vi "MainPanel.vi"() -> ()   [LabVIEW 2017]
uses:
  <vilib>/Native 3D Graph/xcontrol/3DPC_SurfacePlot.xctl
  <vilib>/Simulation/Scripting/Companion Diagram/SimConfigNode/SimParams.ctl
  <vilib>/Simulation/Scripting/Companion Diagram/SimConfigNode/_simSolvers.ctl
  <vilib>/Simulation/Implementation/Shared/SIMSCR Execution Mode.ctl
  <vilib>/Simulation/Param Hierarchy/Typedefs/SIMPH Param Control Actions.ctl
  <vilib>/addons/Control Design/_Model Construction/Model Typedefs.llb/CD Transfer Function Model (MIMO).ctl
  <vilib>/addons/Control Design/_Model Construction/Model Typedefs.llb/CD General Elements.ctl
  <vilib>/addons/Control Design/_Model Construction/Model Typedefs.llb/CD Transfer Function Model (SISO).ctl
  state.ctl
  Mode.ctl
  <vilib>/Simulation/Implementation/Shared/NILVSim_ParamChanged.vi
  <vilib>/Simulation/Implementation/Shared/NILVSIM_BeginStep.vi
  <vilib>/Simulation/Implementation/Shared/NILVSim_Manager.vi
  <vilib>/Utility/error.llb/Clear Errors.vi
  <vilib>/Simulation/Implementation/Shared/NILVSim_FinalizeModel.vi
  <vilib>/Analysis/coordinate.llb/3D Coordinate Conversion (Scalar).vi
  <vilib>/Simulation/Implementation/Shared/SIM Unbundle Sim Info.vi
  <vilib>/Simulation/Implementation/Shared/NILVSim_Initialize.vi
  <vilib>/Simulation/Utility/Implementation/NILVSim Get Time and IsAcceptedStep.vi
  <vilib>/Simulation/Implementation/Shared/SIMSH Read Queue.vi
  <vilib>/Simulation/Implementation/Shared/NILVSim_GetModelError.vi
  <vilib>/Simulation/Implementation/Shared/SIM Bundle Sim Info.vi
  <vilib>/Simulation/Implementation/XNodeFramework/SimXNode/SimX.xnode
  Tension Control.vi
  <vilib>/Simulation/Scripting/Companion Diagram/SimConfigNode/SimDog.xnode
  <vilib>/Analysis/NI_AALPro.lvlib
  <vilib>/Simulation/Implementation/Shared/NI_SIM_Implementation.lvlib
  <vilib>/addons/Control Design/_Model Construction/NI_LinSys_Model Typedefs.lvlib
panel:
  out "Stretch(mm)":dbl(slide) scale=0.0..10.0
  out "Vs":dbl caption="Vs(m/s)" format="%#_4g"
  in  "delay":dbl=100.0 caption="Interval(ms)"
  out "Count":dbl
  out "Rotation":cluster{"Vs":dbl, "Vx":dbl}(graph)
  in  "Forward":bool
  in  "Backward":bool
  in  "Vx":dbl caption="Vx(m/s)" format="%#_5g"
  in  "Deceleration\n  (m/s^-2)":dbl=1.0
  in  "a":dbl=1.0 caption="Acceleration\n (m/s^-2)"
  in  "Range(m)":dbl=5.0 min=0.0
  in  "Layers":dbl format="%#_4g"
  in  "Reverse":bool
  in  "TLimit":dbl=15.0 caption="Max Force(N)" format="%#_4g"
  in  "Tension":bool
  out "Tension\nChart":cluster{"setpoint":dbl, "output y(t)":dbl}(graph)
  in  "F":dbl(slide)=10.0 caption="Set Tension\n (N)" scale=0.0..40.0
  in  "Auto":bool
  in  "Length(m)":dbl=1.5
  in  "Thick":dbl=0.005 caption="Thickness(m)"
  in  "R":dbl(slide)=0.1 caption="Radius(m)" scale=0.0..0.5
  in  "Gap":dbl=0.1 caption="Gap(m)"
  in  "SetSpeed":dbl=100.0 caption="Set Revolution  \n  (RPM)"
  in  "Rapid":bool
  in  "Set X(m)":dbl min=0.0 max=5.0 format="%#_4g"
  in  "Mode":enum32{"Automatic", "Manual"}(radio)
  in  "Home":bool
  in  "Position(m)":dbl(slide) min=0.0 scale=0.0..5.0 scale format="%#_4g"
  out "Trajectory":refnum<class "Base Datatype.lvclass">[](xcontrol)
  in  "Break":bool
  in  "Power":bool
  # "Motion Control Simulation\nBy Xuehui Zhu"
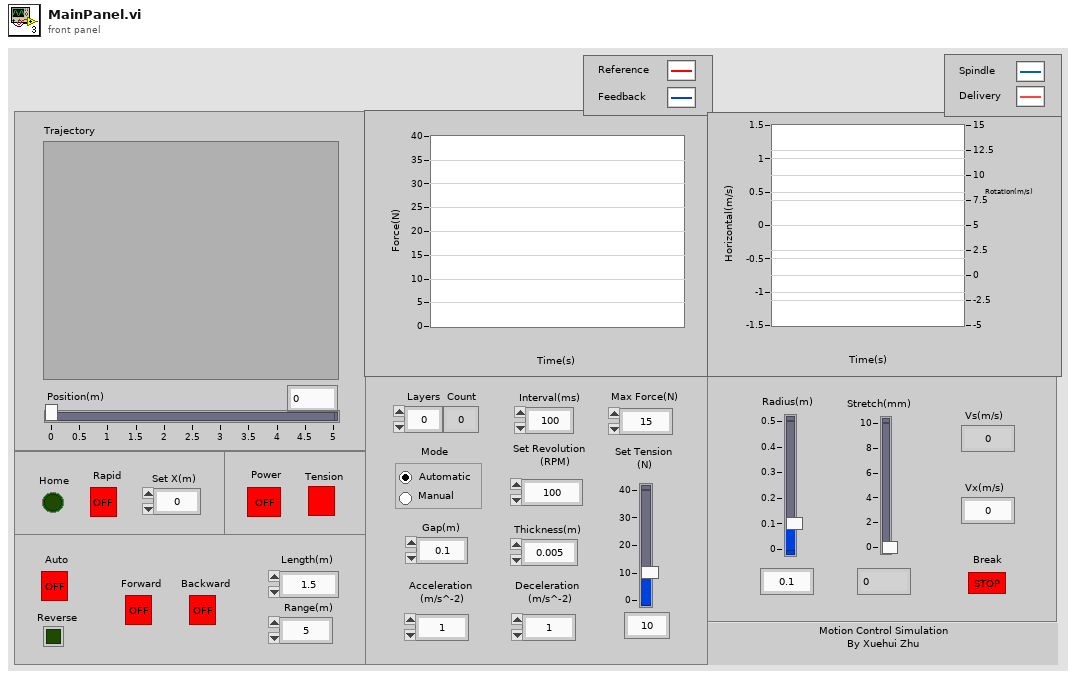
[diagram p1: front panel]
types:
  T1 = enum16{"Simulate to Completion", "Single Time-Step Simulation (Fixed Step Only)"}
  T2 = typedef "SIMSCR Execution Mode.ctl" = enum16{"Simulate to Completion", "Single Time-Step Simulation (Fixed Step Only)"}
  T3 = typedef "SIMPH Param Control Actions.ctl" = enum16{"get params", "set params"}
  T4 = cluster{"proportional gain (Kc)":dbl, "integral time (Ti, min)":dbl, "derivative time (Td, min)":dbl}
  T5 = typedef "NI_LinSys_Model Typedefs.lvlib/CD Transfer Function Model (MIMO).ctl" = cluster{"properties":T6, "transfer function(s)":T7[][]}
  T6 = typedef "NI_LinSys_Model Typedefs.lvlib/CD General Elements.ctl" = cluster{"Model name":string, "Input names":string[], "Output names":string[], "Input Delays":dbl[], "Output Delays":dbl[], "Sampling Time":dbl, "Notes":string}
  T7 = typedef "NI_LinSys_Model Typedefs.lvlib/CD Transfer Function Model (SISO).ctl" = cluster{"Numerator":dbl[], "Denominator":dbl[], "delay":dbl}
  T8 = cluster{"SIMSH Sim Time":dbl, "Gain":cluster{"output":dbl}, "Bundle":cluster{"output cluster":cluster{"setpoint":dbl, "output":dbl}}, "Less?":cluster{"x < y?":bool}, "Transfer Function":cluster{"output y(t)":dbl}, "PID.vi":cluster{"output":dbl}}
  T9 = typedef "SimParams.ctl" = cluster{"Initial Time (s)":dbl, "Final Time (s)":dbl, "Step Size (s)":dbl, "ODE Solver":T10, "Minimum Step Size (s)":dbl, "Maximum Step Size (s)":dbl, "Relative Tolerance":dbl, "Absolute Tolerance":dbl, "Software Timing":bool, "Initial Step Size (s)":dbl, "Automatic Fixed Step Size?":bool, "Automatic Discrete Step Size?":bool, "Discrete Step Size (s)":dbl, "Calculate using Time Step":bool, "Solver Wired?":bool, "Prev.Frm.Expected End":u64, "Prev.Frm.Actual End":u64, "Prev.Frm.Finished Late?":bool, "Prev.Iter.Expected End":u64, "Prev.Iter.Actual End":u64, "Prev.Iter.Finished Late?":bool, "Expected Iteration Start":u64, "Actual Iteration Start":u64, "Expected Frame Start":u64, "Actual Frame Start":u64, "Source Name":string, "Name":string, "Period":i64, "Deadline":i64, "Offset":i64, "Start":i64, "Priority":i32, "Timeout":i32, "Processor":i32, "Mode":enum32{"No Change", "Process missed periods, maintain original phase", "Discard missed periods, maintain original phase", "Process missed periods, ignore original phase", "Discard missed periods, ignore original phase"}, "Wakeup reason":enum32{"Normal", "Aborted", "Asynchronous wakeup", "Timing source error", "Timed loop error", "Timeout"}, "Error":errorcluster, "Source Type":string, "Secondary Source Type":string, "Global End Time":u64, "Global Start Time":u64, "Full Solver Reset":bool, "Execution Mode":T2, "Nan/Inf Check":bool, "Custom Solver Library":string, "Solver Is Variable":bool, "custom solver name":string, "Signal Collection Decimation":u32}
  T10 = typedef "_simSolvers.ctl" = enum16{"Runge-Kutta 1 (Euler)", "Runge-Kutta 2", "Runge-Kutta 3", "Runge-Kutta 4", "Runge-Kutta 23 (variable)", "Runge-Kutta 45 (variable)", "BDF (variable)", "Adams-Moulton (variable)", "Rosenbrock (variable)", "Discrete States Only", "SDIRK 4 (variable)", "Radau 5 (variable)", "Radau 9 (variable)", "Radau 13 (variable)", "Radau [Variable Order] (variable)", "Gear's Method (variable)", "Linearizer", "State Query", "Trim Eval", "Custom Solver"}
  T11 = typedef "state.ctl" = enum16{"Wait", "Forward", "Backward"}
  T12 = typedef "Mode.ctl" = enum32{"Automatic", "Manual"}
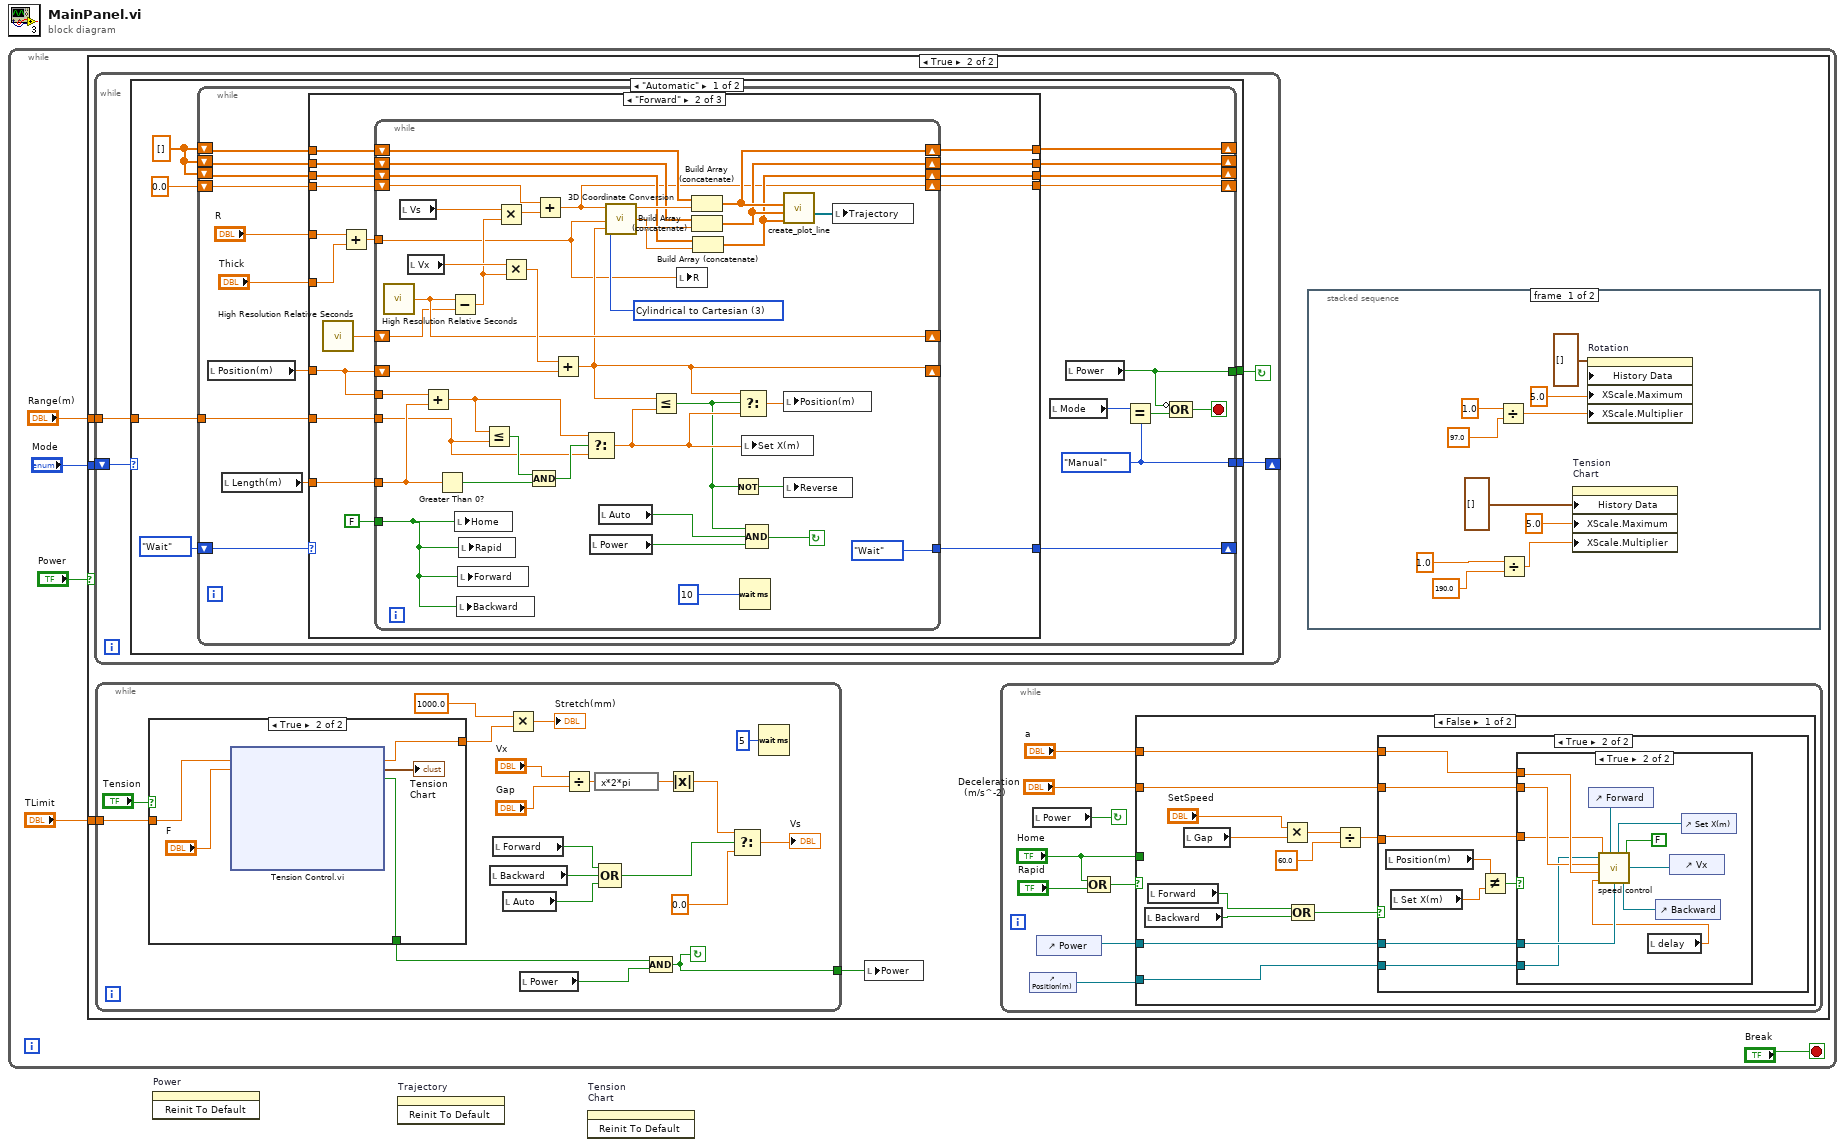
[diagram p0: block diagram]
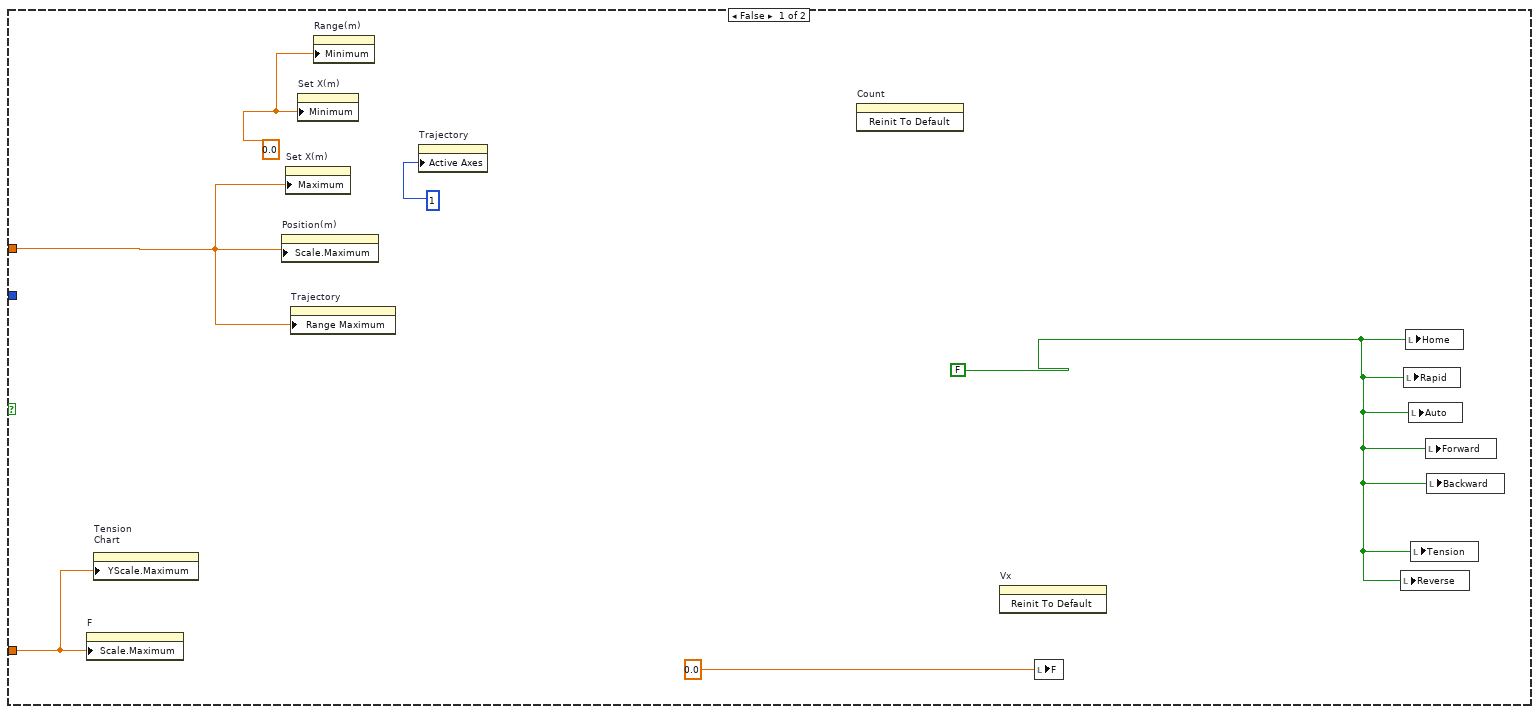
[diagram p2: hidden frame]
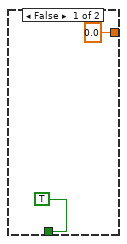
[diagram p3: hidden frame]
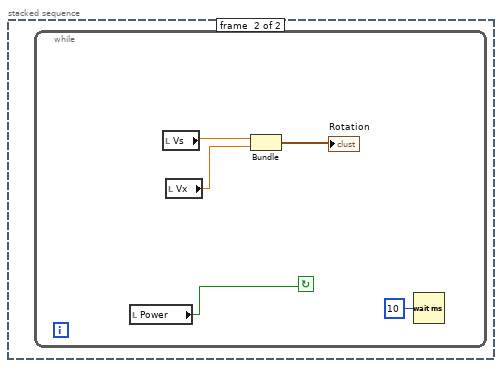
[diagram p4: hidden frame]
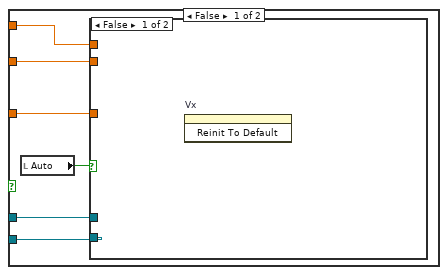
[diagram p5: hidden frame]
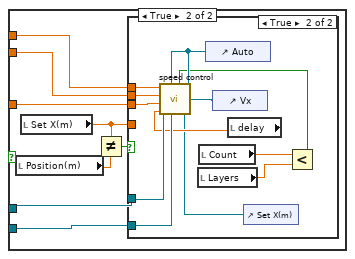
[diagram p6: hidden frame]
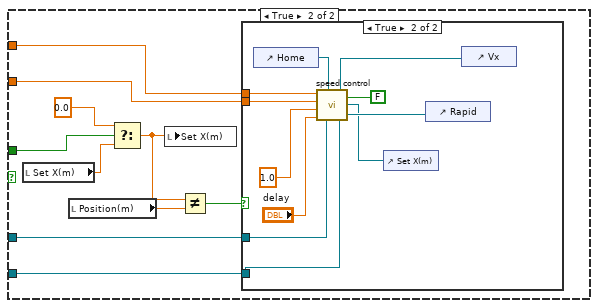
[diagram p9: hidden frame]
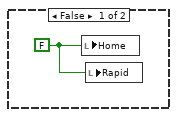
[diagram p10: hidden frame]
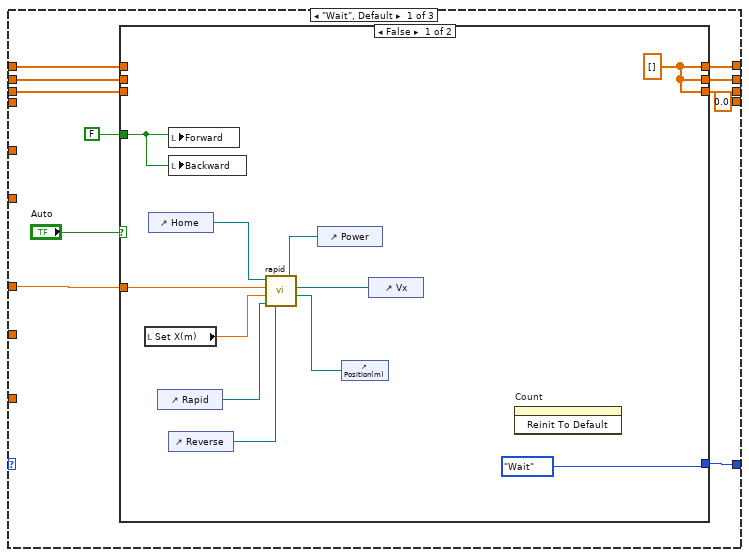
[diagram p11: hidden frame]
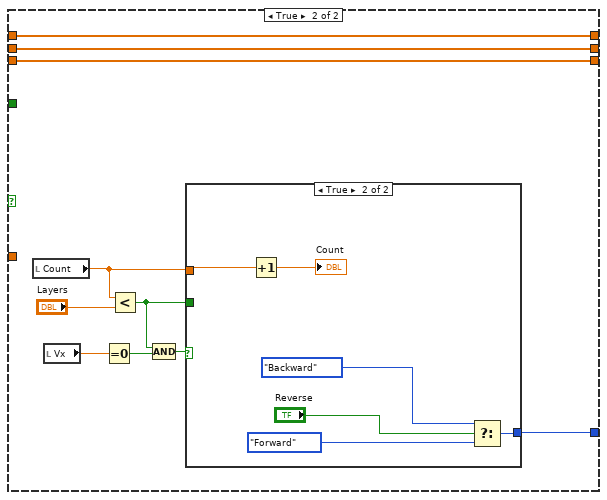
[diagram p12: hidden frame]
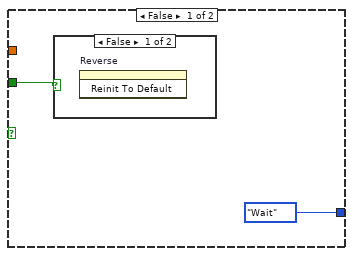
[diagram p13: hidden frame]
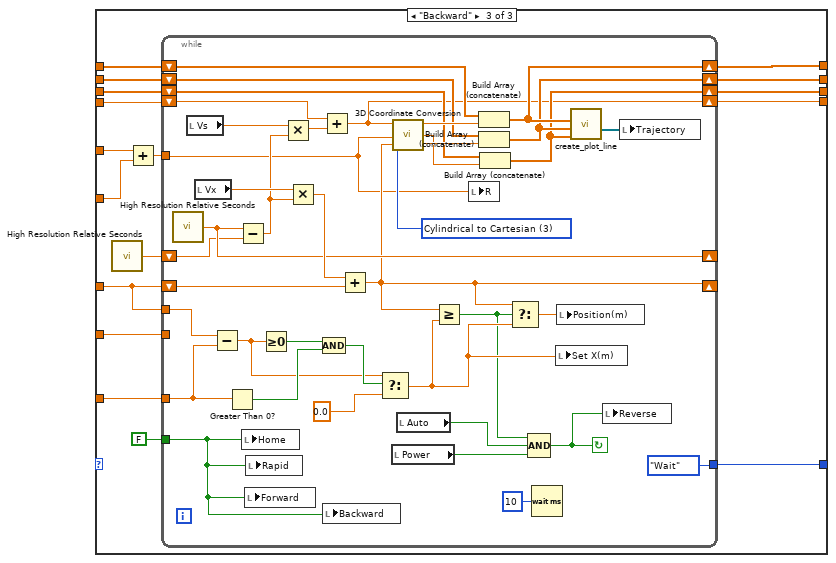
[diagram p15: hidden frame]
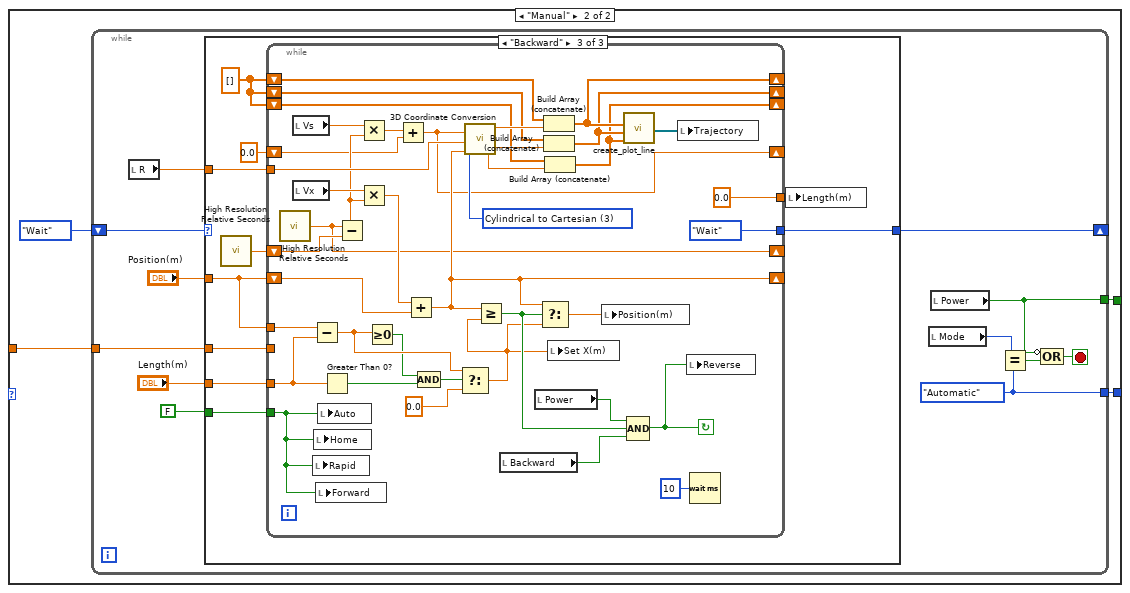
[diagram p16: hidden frame]
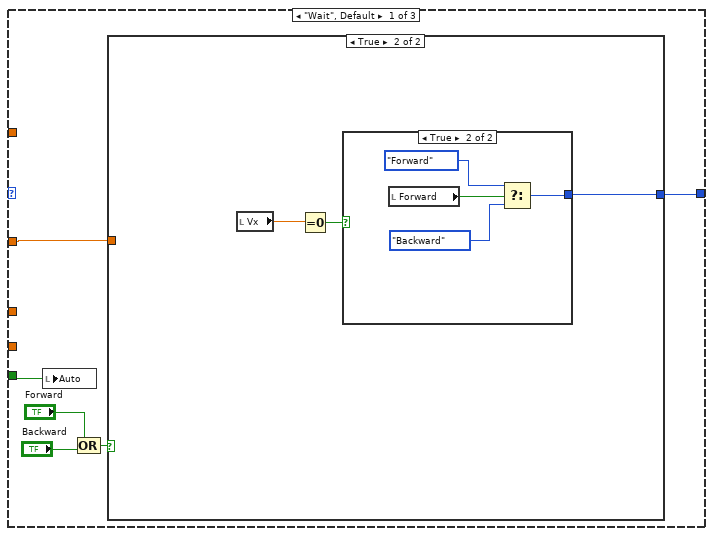
[diagram p17: hidden frame]
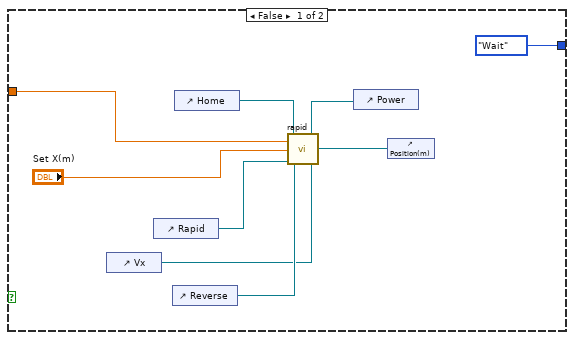
[diagram p18: hidden frame]
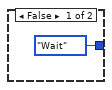
[diagram p19: hidden frame]
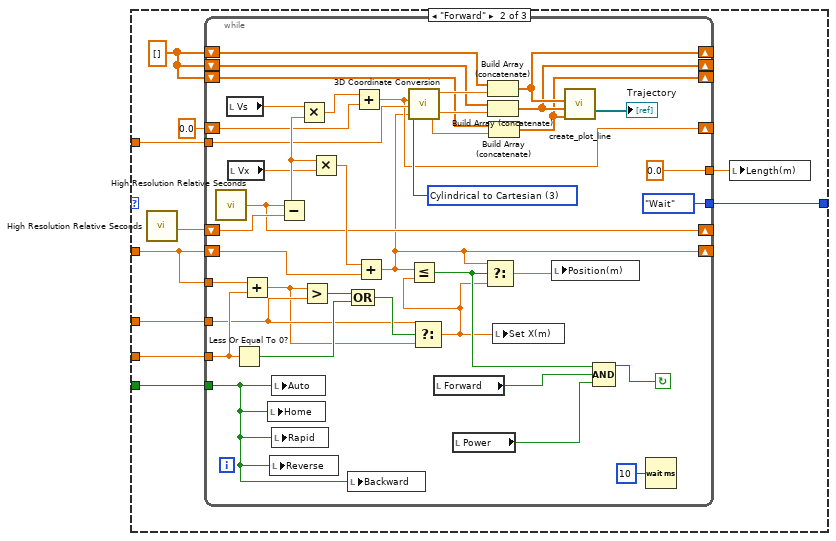
[diagram p20: hidden frame]
diagram:
  n1 = while {
    stop <- "Break" stop-if-true
    n2 = case shown="True" "Power" {
      tunnel: "Range(m)" -> [w8 w14]
      tunnel: "TLimit" -> [w9 w12]
      tunnel: "Mode" -> [_ w13]
      frame False {
        w7 = 0.0 ("Data Entry Limits:Minimum")
        w6 = FALSE ("zero")
        n3 = property on="F" class="Slide (strict)"("Scale.Maximum"=w9) -> ()  [unwired: 2 in, 2 out]
        n4 = property on="Tension\nChart" class="WFChart (strict)"("YScale.Maximum"=w9) -> ()  [unwired: 2 in, 2 out]
        n5 = property on="Position(m)" class="Slide (strict)"("Scale.Maximum"=w8) -> ()  [unwired: 2 in, 2 out]
        n6 = property on="Set X(m)" class="DigNum (strict)"("Maximum"=w8) -> ()  [unwired: 2 in, 2 out]
        n7 = property on="Trajectory" class="LabVIEW 3D Graph (strict)"("Range Maximum"=w8) -> ()  [unwired: 2 in, 2 out]
        n8 = property on="Set X(m)" class="DigNum (strict)"("Minimum"=w7) -> ()  [unwired: 2 in, 2 out]
        n9 = property on="Range(m)" class="DigNum (strict)"("Minimum"=w7) -> ()  [unwired: 2 in, 2 out]
        n10 = property on="Trajectory" class="LabVIEW 3D Graph (strict)"("Active Axes"=1 ("Axes:Active Axis")) -> ()  [unwired: 2 in, 2 out]
        n11 = invoke on="Count" class="DigNum (strict)" method="Reinit To Default"() -> ()  [unwired: 3 in, 3 out]
        n12 = invoke on="Vx" class="DigNum (strict)" method="Reinit To Default"() -> ()  [unwired: 3 in, 3 out]
        n13 = local write "F"(0.0 ("Set Force \n     (N)")) -> ()
        n14 = local write "Reverse"(w6) -> ()
        n15 = local write "Rapid"(w6) -> ()
        n16 = local write "Home"(w6) -> ()
        n17 = local write "Auto"(w6) -> ()
        n18 = local write "Tension"(w6) -> ()
        n19 = local write "Forward"(w6) -> ()
        n20 = local write "Backward"(w6) -> ()
      }
      frame True {
        n21 = while {
          shift-right: [w424] -> _
          shift-left: w13 -> [w423]
          tunnel: w14 -> [w422]
          stop <- w421 continue-if-true
          n22 = case shown="\"Automatic\"" w423 {
            tunnel: w422 -> [w428 w606]
            tunnel: [w427 w605] -> w424
            tunnel: [w426 w604] -> w421
            frame "Automatic" {
              w429 = dbl[] []
              n23 = while {
                shift-right: [w449] -> _
                shift-left: state."Wait" ("Enum") -> [w450]
                shift-right: [w446] -> _
                shift-left: w429 -> [w443]
                shift-right: [w445] -> _
                shift-left: w429 -> [w442]
                shift-right: [w444] -> _
                shift-left: w429 -> [w441]
                tunnel: w428 -> [w439]
                tunnel: [w437] -> w427
                tunnel: [w434] -> w426
                shift-right: [w431] -> _
                shift-left: 0.0 -> [w432]
                stop <- w435 stop-if-true
                w437 = Mode."Manual" ("Mode")
                n24 = local read "Position(m)"() -> (w448:dbl)
                n25 = local read "Length(m)"() -> (w433:dbl)
                n26 = case shown="\"Forward\"" w450 {
                  tunnel: "R" -> [_ w494 w551]
                  tunnel: [w460 w506 w563] -> w449
                  tunnel: w448 -> [w453 w496 w553]
                  tunnel: w433 -> [_ w507 w564]
                  tunnel: [w458 w504 w561] -> w446
                  tunnel: [w456 w503 w560] -> w445
                  tunnel: [w454 w502 w559] -> w444
                  tunnel: w443 -> [w459 w501 w558]
                  tunnel: w442 -> [w457 w500 w557]
                  tunnel: w441 -> [w455 w499 w556]
                  tunnel: w439 -> [_ w497 w554]
                  tunnel: "Thick" -> [_ w495 w552]
                  tunnel: w432 -> [_ w492 w549]
                  tunnel: [0.0 w491 w548] -> w431
                  frame "Wait", Default {
                    n27 = case shown="False" "Auto" {
                      tunnel: [state."Wait" ("Enum") w482] -> w460
                      tunnel: w459 -> [_ w477]
                      tunnel: [w463 w477] -> w458
                      tunnel: w457 -> [_ w476]
                      tunnel: [w463 w476] -> w456
                      tunnel: w455 -> [_ w475]
                      tunnel: [w463 w475] -> w454
                      tunnel: w453 -> [w464 _]
                      tunnel: FALSE -> [w462 _]
                      frame False {
                        w463 = dbl[] []
                        n28 = local read "Set X(m)"() -> (w470:dbl)
                        n29 = control-ref of="Home"() -> (w471:refnum<vi>)
                        n30 = control-ref of="Rapid"() -> (w469:refnum<vi>)
                        n31 = local write "Forward"(w462) -> ()
                        n32 = local write "Backward"(w462) -> ()
                        n33 = control-ref of="Reverse"() -> (w466:refnum<vi>)
                        n34 = control-ref of="Power"() -> (w467:refnum<vi>)
                        n35 = control-ref of="Position(m)"() -> (w468:refnum<vi>)
                        n36 = control-ref of="Vx"() -> (w465:refnum<vi>)
                        n37 = call "rapid.vi"("Speed"=w465, "positon"=w468, "Reverse"=w466, "Power"=w467, "Rapid"=w469, "Set x"=w470, "Input"=w464, "Zero"=w471) -> ()
                        n38 = invoke on="Count" class="DigNum (strict)" method="Reinit To Default"() -> ()  [unwired: 3 in, 3 out]
                      }
                      frame True {
                        n39 = local read "Count"() -> (w478:dbl)
                        n40 = local read "Vx"() -> (w481:dbl)
                        n41 = Equal To 0?(x=w481) -> (x = 0?=w474:bool)
                        n42 = Less?(x=w478, y="Layers") -> (x < y?=w473:bool)
                        n43 = Compound Arithmetic op=AND(w473, w474) -> (w480:bool)
                        n44 = case shown="True" w480 {
                          tunnel: [state."Wait" ("Enum") w488] -> w482
                          tunnel: w478 -> [_ w486]
                          tunnel: w473 -> [w483 _]
                          frame False {
                            n45 = case shown="False" w483 {
                              frame False {
                                n46 = invoke on="Reverse" class="Bool (strict)" method="Reinit To Default"() -> ()  [unwired: 3 in, 3 out]
                              }
                              frame True {
                              }
                            }
                          }
                          frame True {
                            n47 = Increment(x=w486) -> (x+1=→"Count":dbl)
                            n48 = Select(t=state."Backward" ("Enum"), s="Reverse", f=state."Forward" ("Enum")) -> (s? t:f=w488:T11)
                          }
                        }
                      }
                    }
                  }
                  frame "Forward" {
                    n49 = call <vilib>:"High Resolution Relative Seconds.vi"() -> ("relative seconds"=w498:dbl)
                    n50 = Add(x=w494, y=w495) -> (x+y=w493:dbl)
                    n51 = while {
                      tunnel: w507 -> [w528]
                      tunnel: [state."Wait" ("Enum")] -> w506
                      shift-right: [w543] -> w504
                      shift-left: w501 -> [w540]
                      shift-right: [w542] -> w503
                      shift-left: w500 -> [w539]
                      shift-right: [w541] -> w502
                      shift-left: w499 -> [w538]
                      tunnel: FALSE -> [w514]
                      tunnel: w497 -> [w510]
                      shift-right: [w531] -> _
                      shift-left: w498 -> [w530]
                      shift-right: [w525] -> _
                      shift-left: w496 -> [w537]
                      tunnel: w496 -> [w529]
                      tunnel: w493 -> [w520]
                      shift-right: [w516] -> w491
                      shift-left: w492 -> [w518]
                      stop <- w509 continue-if-true
                      w547 = u16 3 items=["Cartesian to Spherical", "Spherical to Cartesian", "Cartesian to Cylindrical", "Cylindrical to Cartesian", "Spherical to Cylindrical", "Cylindrical to Spherical"] ("conversion type")
                      n52 = call <vilib>:"High Resolution Relative Seconds.vi"() -> ("relative seconds"=w531:dbl)
                      n53 = local read "Vs"() -> (w519:dbl)
                      n54 = local read "Vx"() -> (w522:dbl)
                      n55 = Add(x=w529, y=w528) -> (x+y=w524:dbl)
                      n56 = Greater Than 0?(x=w528) -> (x > 0?=w527:bool)
                      n57 = Subtract(x=w531, y=w530) -> (x-y=w521:dbl)
                      n58 = local write "Home"(w514) -> ()
                      n59 = local write "Backward"(w514) -> ()
                      n60 = local write "Forward"(w514) -> ()
                      n61 = local write "Rapid"(w514) -> ()
                      n62 = Less Or Equal?(x=w524, y=w510) -> (x <= y?=w526:bool)
                      n63 = Multiply(x=w519, y=w521) -> (x*y=w517:dbl)
                      n64 = Multiply(x=w522, y=w521) -> (x*y=w532:dbl)
                      n65 = Compound Arithmetic op=AND(w526, w527) -> (w513:bool)
                      n66 = Add(x=w518, y=w517) -> (x+y=w516:dbl)
                      n67 = Add(x=w532, y=w537) -> (x+y=w525:dbl)
                      n68 = Select(t=w524, s=w513, f=w510) -> (s? t:f=w523:dbl)
                      n69 = local read "Power"() -> (w535:bool)
                      n70 = local read "Auto"() -> (w536:bool)
                      n71 = call-poly <vilib>:"3D Coordinate Conversion.vi"("conversion type"=w547, "axis 3"=w525, "axis 2"=w516, "axis 1"=w520) -> ("axis 3 out"=w546:dbl, "axis 2 out"=w544:dbl, "axis 1 out"=w545:dbl)  [unwired: 4 in, 1 out]
                      n72 = Less Or Equal?(x=w525, y=w523) -> (x <= y?=w508:bool)
                      n73 = local write "R"(w520) -> ()
                      n74 = Build Array (concatenate)(w540, w544) -> (w543:dbl[])
                      n75 = Build Array (concatenate)(w539, w546) -> (w542:dbl[])
                      n76 = Build Array (concatenate)(w538, w545) -> (w541:dbl[])
                      n77 = Not(x=w508) -> (.not. x?=w511:bool)
                      n78 = Select(t=w525, s=w508, f=w523) -> (s? t:f=w533:dbl)
                      n79 = Wait (ms)(milliseconds to wait=u32 10) -> ()  [unwired: 1 out]
                      n80 = local write "Set X(m)"(w523) -> ()
                      n81 = Compound Arithmetic op=AND(w508, w536, w535) -> (w509:bool)
                      n82 = call <vilib>:"create_plot_line.vi"("z vector"=w541, "y vector"=w542, "x vector"=w543) -> ("plots out"=w534:refnum<class "Base Datatype.lvclass">[])  [unwired: 2 in, 6 out]
                      n83 = local write "Position(m)"(w533) -> ()
                      n84 = local write "Reverse"(w511) -> ()
                      n85 = local write "Trajectory"(w534) -> ()
                    }
                  }
                  frame "Backward" {
                    n86 = call <vilib>:"High Resolution Relative Seconds.vi"() -> ("relative seconds"=w555:dbl)
                    n87 = Add(x=w551, y=w552) -> (x+y=w550:dbl)
                    n88 = while {
                      tunnel: w564 -> [w584]
                      tunnel: [state."Wait" ("Enum")] -> w563
                      shift-right: [w599] -> w561
                      shift-left: w558 -> [w596]
                      shift-right: [w598] -> w560
                      shift-left: w557 -> [w595]
                      shift-right: [w597] -> w559
                      shift-left: w556 -> [w594]
                      tunnel: FALSE -> [w568]
                      tunnel: w554 -> [_]
                      shift-right: [w587] -> _
                      shift-left: w555 -> [w586]
                      shift-right: [w581] -> _
                      shift-left: w553 -> [w593]
                      tunnel: w553 -> [w585]
                      tunnel: w550 -> [w575]
                      shift-right: [w571] -> w548
                      shift-left: w549 -> [w573]
                      stop <- w565 continue-if-true
                      w603 = u16 3 items=["Cartesian to Spherical", "Spherical to Cartesian", "Cartesian to Cylindrical", "Cylindrical to Cartesian", "Spherical to Cylindrical", "Cylindrical to Spherical"] ("conversion type")
                      n89 = call <vilib>:"High Resolution Relative Seconds.vi"() -> ("relative seconds"=w587:dbl)
                      n90 = local read "Vs"() -> (w574:dbl)
                      n91 = local read "Vx"() -> (w577:dbl)
                      n92 = Subtract(x=w585, y=w584) -> (x-y=w569:dbl)
                      n93 = Greater Than 0?(x=w584) -> (x > 0?=w583:bool)
                      n94 = Subtract(x=w587, y=w586) -> (x-y=w576:dbl)
                      n95 = local write "Home"(w568) -> ()
                      n96 = local write "Forward"(w568) -> ()
                      n97 = local write "Rapid"(w568) -> ()
                      n98 = Greater Or Equal To 0?(x=w569) -> (x >= 0?=w582:bool)
                      n99 = Multiply(x=w574, y=w576) -> (x*y=w572:dbl)
                      n100 = Multiply(x=w577, y=w576) -> (x*y=w588:dbl)
                      n101 = Add(x=w573, y=w572) -> (x+y=w571:dbl)
                      n102 = Compound Arithmetic op=AND(w582, w583) -> (w578:bool)
                      n103 = local write "Backward"(w568) -> ()
                      n104 = Add(x=w588, y=w593) -> (x+y=w581:dbl)
                      n105 = Select(t=w569, s=w578, f=0.0) -> (s? t:f=w579:dbl)
                      n106 = local read "Power"() -> (w591:bool)
                      n107 = call-poly <vilib>:"3D Coordinate Conversion.vi"("conversion type"=w603, "axis 3"=w581, "axis 2"=w571, "axis 1"=w575) -> ("axis 3 out"=w602:dbl, "axis 2 out"=w600:dbl, "axis 1 out"=w601:dbl)  [unwired: 4 in, 1 out]
                      n108 = local read "Auto"() -> (w592:bool)
                      n109 = Greater Or Equal?(x=w581, y=w579) -> (x >= y?=w566:bool)
                      n110 = local write "R"(w575) -> ()
                      n111 = Build Array (concatenate)(w596, w600) -> (w599:dbl[])
                      n112 = Build Array (concatenate)(w595, w602) -> (w598:dbl[])
                      n113 = Build Array (concatenate)(w594, w601) -> (w597:dbl[])
                      n114 = Select(t=w581, s=w566, f=w579) -> (s? t:f=w589:dbl)
                      n115 = Compound Arithmetic op=AND(w566, w592, w591) -> (w565:bool)
                      n116 = Wait (ms)(milliseconds to wait=u32 10) -> ()  [unwired: 1 out]
                      n117 = local write "Set X(m)"(w579) -> ()
                      n118 = local write "Position(m)"(w589) -> ()
                      n119 = call <vilib>:"create_plot_line.vi"("z vector"=w597, "y vector"=w598, "x vector"=w599) -> ("plots out"=w590:refnum<class "Base Datatype.lvclass">[])  [unwired: 2 in, 6 out]
                      n120 = local write "Reverse"(w565) -> ()
                      n121 = local write "Trajectory"(w590) -> ()
                    }
                  }
                }
                n122 = local read "Mode"() -> (w447:enum32{"Automatic", "Manual"})
                n123 = local read "Power"() -> (w434:bool)
                n124 = Equal?(x=w447, y=w437) -> (x = y?=w436:bool)
                n125 = Compound Arithmetic op=OR(invert w434, w436) -> (w435:bool)
              }
            }
            frame "Manual" {
              n126 = while {
                shift-right: [w618] -> _
                shift-left: state."Wait" ("Enum") -> [w619]
                tunnel: w606 -> [w608]
                tunnel: [w612] -> w605
                tunnel: [w609] -> w604
                stop <- w610 stop-if-true
                w612 = Mode."Automatic" ("Mode")
                n127 = local read "R"() -> (w613:dbl)
                n128 = case shown="\"Backward\"" w619 {
                  tunnel: "Length(m)" -> [_ w652 w701]
                  tunnel: FALSE -> [w620 w651 w700]
                  tunnel: w613 -> [_ w650 w699]
                  tunnel: [w623 w649 w698] -> w618
                  tunnel: "Position(m)" -> [w625 w643 w694]
                  tunnel: w608 -> [_ w646 w695]
                  frame "Wait", Default {
                    n129 = local write "Auto"(w620) -> ()
                    n130 = Compound Arithmetic op=OR("Forward", "Backward") -> (w624:bool)
                    n131 = case shown="True" w624 {
                      tunnel: w625 -> [w629 _]
                      tunnel: [state."Wait" ("Enum") w637] -> w623
                      frame False {
                        n132 = control-ref of="Vx"() -> (w627:refnum<vi>)
                        n133 = control-ref of="Rapid"() -> (w632:refnum<vi>)
                        n134 = control-ref of="Reverse"() -> (w633:refnum<vi>)
                        n135 = control-ref of="Home"() -> (w634:refnum<vi>)
                        n136 = control-ref of="Power"() -> (w631:refnum<vi>)
                        n137 = control-ref of="Position(m)"() -> (w628:refnum<vi>)
                        n138 = call "rapid.vi"("Speed"=w627, "positon"=w628, "Reverse"=w633, "Power"=w631, "Rapid"=w632, "Set x"="Set X(m)", "Input"=w629, "Zero"=w634) -> ()
                      }
                      frame True {
                        n139 = local read "Vx"() -> (w636:dbl)
                        n140 = Equal To 0?(x=w636) -> (x = 0?=w635:bool)
                        n141 = case shown="True" w635 {
                          tunnel: [state."Wait" ("Enum") w642] -> w637
                          frame False {
                          }
                          frame True {
                            n142 = local read "Forward"() -> (w641:bool)
                            n143 = Select(t=state."Forward" ("Enum"), s=w641, f=state."Backward" ("Enum")) -> (s? t:f=w642:T11)
                          }
                        }
                      }
                    }
                  }
                  frame "Forward" {
                    w647 = dbl[] []
                    n144 = call <vilib>:"High Resolution Relative Seconds.vi"() -> ("relative seconds"=w645:dbl)
                    n145 = while {
                      tunnel: w650 -> [w686]
                      tunnel: w652 -> [w661]
                      tunnel: w651 -> [w655]
                      tunnel: [state."Wait" ("Enum")] -> w649
                      tunnel: [0.0 ("Length(m)")] -> w648
                      shift-right: [w683] -> _
                      shift-left: w647 -> [w680]
                      shift-right: [w682] -> _
                      shift-left: w647 -> [w679]
                      shift-right: [w681] -> _
                      shift-left: w647 -> [w678]
                      tunnel: w646 -> [w660]
                      shift-right: [w670] -> _
                      shift-left: w645 -> [w671]
                      shift-right: [w665] -> _
                      shift-left: w643 -> [w669]
                      shift-right: [w666] -> _
                      shift-left: 0.0 -> [w667]
                      tunnel: w643 -> [w662]
                      stop <- w656 continue-if-true
                      w692 = u16 3 items=["Cartesian to Spherical", "Spherical to Cartesian", "Cartesian to Cylindrical", "Cylindrical to Cartesian", "Spherical to Cylindrical", "Cylindrical to Spherical"] ("conversion type")
                      n146 = call <vilib>:"High Resolution Relative Seconds.vi"() -> ("relative seconds"=w670:dbl)
                      n147 = local read "Vs"() -> (w663:dbl)
                      n148 = local read "Vx"() -> (w664:dbl)
                      n149 = Less Or Equal To 0?(x=w661) -> (x <= 0?=w674:bool)
                      n150 = Add(x=w662, y=w661) -> (x+y=w659:dbl)
                      n151 = local write "Home"(w655) -> ()
                      n152 = local write "Reverse"(w655) -> ()
                      n153 = local write "Auto"(w655) -> ()
                      n154 = local write "Rapid"(w655) -> ()
                      n155 = Subtract(x=w670, y=w671) -> (x-y=w688:dbl)
                      n156 = Multiply(x=w663, y=w688) -> (x*y=w668:dbl)
                      n157 = Greater?(x=w659, y=w660) -> (0:w673:bool)
                      n158 = Multiply(x=w688, y=w664) -> (x*y=w675:dbl)
                      n159 = local write "Backward"(w655) -> ()
                      n160 = Compound Arithmetic op=OR(w673, w674) -> (w672:bool)
                      n161 = Add(x=w668, y=w667) -> (x+y=w666:dbl)
                      n162 = Add(x=w675, y=w669) -> (x+y=w665:dbl)
                      n163 = call-poly <vilib>:"3D Coordinate Conversion.vi"("conversion type"=w692, "axis 3"=w665, "axis 2"=w666, "axis 1"=w686) -> ("axis 3 out"=w690:dbl, "axis 2 out"=w685:dbl, "axis 1 out"=w689:dbl)  [unwired: 4 in, 1 out]
                      n164 = Select(t=w660, s=w672, f=w659) -> (s? t:f=w658:dbl)
                      n165 = Less Or Equal?(x=w665, y=w658) -> (x <= y?=w677:bool)
                      n166 = local read "Forward"() -> (w653:bool)
                      n167 = local read "Power"() -> (w654:bool)
                      n168 = Select(t=w665, s=w677, f=w658) -> (s? t:f=w676:dbl)
                      n169 = Build Array (concatenate)(w680, w685) -> (w683:dbl[])
                      n170 = Build Array (concatenate)(w679, w690) -> (w682:dbl[])
                      n171 = Build Array (concatenate)(w678, w689) -> (w681:dbl[])
                      n172 = local write "Set X(m)"(w658) -> ()
                      n173 = local write "Position(m)"(w676) -> ()
                      n174 = call <vilib>:"create_plot_line.vi"("z vector"=w681, "y vector"=w682, "x vector"=w683) -> ("plots out"=→"Trajectory":refnum<class "Base Datatype.lvclass">[])  [unwired: 2 in, 6 out]
                      n175 = Compound Arithmetic op=AND(w677, w653, w654) -> (w656:bool)
                      n176 = Wait (ms)(milliseconds to wait=u32 10) -> ()  [unwired: 1 out]
                    }
                    n177 = local write "Length(m)"(w648) -> ()
                  }
                  frame "Backward" {
                    w696 = dbl[] []
                    n178 = call <vilib>:"High Resolution Relative Seconds.vi"() -> ("relative seconds"=w702:dbl)
                    n179 = while {
                      tunnel: w699 -> [w738]
                      tunnel: w701 -> [w710]
                      tunnel: w700 -> [w704]
                      tunnel: [state."Wait" ("Enum")] -> w698
                      tunnel: [0.0 ("Length(m)")] -> w697
                      shift-right: [w734] -> _
                      shift-left: w696 -> [w731]
                      shift-right: [w733] -> _
                      shift-left: w696 -> [w730]
                      shift-right: [w732] -> _
                      shift-left: w696 -> [w729]
                      tunnel: w695 -> [_]
                      shift-right: [w711] -> _
                      shift-left: w702 -> [w722]
                      shift-right: [w717] -> _
                      shift-left: w694 -> [w723]
                      tunnel: w694 -> [w719]
                      shift-right: [w712] -> _
                      shift-left: 0.0 -> [w713]
                      stop <- w725 continue-if-true
                      w742 = u16 3 items=["Cartesian to Spherical", "Spherical to Cartesian", "Cartesian to Cylindrical", "Cylindrical to Cartesian", "Spherical to Cylindrical", "Cylindrical to Spherical"] ("conversion type")
                      n180 = call <vilib>:"High Resolution Relative Seconds.vi"() -> ("relative seconds"=w711:dbl)
                      n181 = local read "Vs"() -> (w715:dbl)
                      n182 = local read "Vx"() -> (w721:dbl)
                      n183 = Subtract(x=w719, y=w710) -> (x-y=w718:dbl)
                      n184 = local write "Rapid"(w704) -> ()
                      n185 = local write "Home"(w704) -> ()
                      n186 = local write "Forward"(w704) -> ()
                      n187 = local write "Auto"(w704) -> ()
                      n188 = Greater Than 0?(x=w710) -> (x > 0?=w708:bool)
                      n189 = Subtract(x=w711, y=w722) -> (x-y=w720:dbl)
                      n190 = Multiply(x=w715, y=w720) -> (x*y=w714:dbl)
                      n191 = Multiply(x=w721, y=w720) -> (x*y=w724:dbl)
                      n192 = Greater Or Equal To 0?(x=w718) -> (x >= 0?=w709:bool)
                      n193 = Add(x=w714, y=w713) -> (x+y=w712:dbl)
                      n194 = Add(x=w724, y=w723) -> (x+y=w717:dbl)
                      n195 = Compound Arithmetic op=AND(w709, w708) -> (w707:bool)
                      n196 = Select(t=w718, s=w707, f=0.0) -> (s? t:f=w716:dbl)
                      n197 = call-poly <vilib>:"3D Coordinate Conversion.vi"("conversion type"=w742, "axis 3"=w717, "axis 2"=w712, "axis 1"=w738) -> ("axis 3 out"=w741:dbl, "axis 2 out"=w737:dbl, "axis 1 out"=w740:dbl)  [unwired: 4 in, 1 out]
                      n198 = Greater Or Equal?(x=w717, y=w716) -> (x >= y?=w727:bool)
                      n199 = local read "Backward"() -> (w703:bool)
                      n200 = local read "Power"() -> (w735:bool)
                      n201 = Select(t=w717, s=w727, f=w716) -> (s? t:f=w726:dbl)
                      n202 = Build Array (concatenate)(w731, w737) -> (w734:dbl[])
                      n203 = Build Array (concatenate)(w730, w741) -> (w733:dbl[])
                      n204 = Build Array (concatenate)(w729, w740) -> (w732:dbl[])
                      n205 = local write "Set X(m)"(w716) -> ()
                      n206 = local write "Position(m)"(w726) -> ()
                      n207 = call <vilib>:"create_plot_line.vi"("z vector"=w732, "y vector"=w733, "x vector"=w734) -> ("plots out"=w728:refnum<class "Base Datatype.lvclass">[])  [unwired: 2 in, 6 out]
                      n208 = Compound Arithmetic op=AND(w735, w727, w703) -> (w725:bool)
                      n209 = local write "Trajectory"(w728) -> ()
                      n210 = local write "Reverse"(w725) -> ()
                      n211 = Wait (ms)(milliseconds to wait=u32 10) -> ()  [unwired: 1 out]
                    }
                    n212 = local write "Length(m)"(w697) -> ()
                  }
                }
                n213 = local read "Mode"() -> (w615:enum32{"Automatic", "Manual"})
                n214 = local read "Power"() -> (w609:bool)
                n215 = Equal?(x=w615, y=w612) -> (x = y?=w611:bool)
                n216 = Compound Arithmetic op=OR(invert w609, w611) -> (w610:bool)
              }
            }
          }
        }
        n217 = while {
          tunnel: [w33] -> w15
          tunnel: w12 -> [w32]
          stop <- w33 continue-if-true
          n218 = case shown="True" "Tension" {
            tunnel: [TRUE ("Warning") w40] -> w34
            tunnel: w32 -> [_ w42]
            tunnel: [0.0 ("Numeric") w38] -> w18
            frame False {
            }
            frame True {
              n219 = xnode "Tension Control.vi"("Tension Limit(N)"=w42, "setpoint"="F") -> ("Numeric"=w38:dbl, "Waveform Chart"=→"Tension\nChart":cluster{"setpoint":dbl, "output y(t)":dbl}, "Warning"=w40:bool)  [unwired: 2 in, 1 out]
            }
          }
          n220 = local read "Backward"() -> (w24:bool)
          n221 = local read "Forward"() -> (w25:bool)
          n222 = local read "Auto"() -> (w23:bool)
          n223 = Multiply(x=1000.0, y=w18) -> (x*y=→"Stretch(mm)":dbl)
          n224 = local read "Power"() -> (w35:bool)
          n225 = Divide(x="Vx", y="Gap") -> (x/y=w28:dbl)
          n226 = expression code="x*2*pi"(w28) -> (w27:dbl)
          n227 = Compound Arithmetic op=OR(w25, w24, w23) -> (w22:bool)
          n228 = Compound Arithmetic op=AND(w34, w35) -> (w33:bool)
          n229 = Absolute Value(x=w27) -> (abs(x)=w26:dbl)
          n230 = Select(t=w26, s=w22, f=0.0) -> (s? t:f=→"Vs":dbl)
          n231 = Wait (ms)(milliseconds to wait=u32 5) -> ()  [unwired: 1 out]
        }
        n232 = local write "Power"(w15) -> ()
        n233 = while {
          stop <- w339 continue-if-true
          n234 = control-ref of="Position(m)"() -> (w334:refnum<vi>)
          n235 = local read "Power"() -> (w339:bool)
          n236 = control-ref of="Power"() -> (w335:refnum<vi>)
          n237 = Compound Arithmetic op=OR("Home", "Rapid") -> (w337:bool)
          n238 = case shown="False" w337 {
            tunnel: "a" -> [w352 w408]
            tunnel: "Deceleration\n  (m/s^-2)" -> [w351 w407]
            tunnel: "Home" -> [_ w405]
            tunnel: w335 -> [w350 w404]
            tunnel: w334 -> [w349 w403]
            frame False {
              n239 = local read "Backward"() -> (w353:bool)
              n240 = local read "Forward"() -> (w342:bool)
              n241 = local read "Gap"() -> (w344:dbl)
              n242 = Multiply(x="SetSpeed", y=w344) -> (x*y=w347:dbl)
              n243 = Compound Arithmetic op=OR(w342, w353) -> (w348:bool)
              n244 = Divide(x=w347, y=60.0) -> (x/y=w345:dbl)
              n245 = case shown="True" w348 {
                tunnel: w352 -> [w358 w387]
                tunnel: w351 -> [w357 w386]
                tunnel: w350 -> [w355 w385]
                tunnel: w349 -> [w354 w384]
                tunnel: w345 -> [w356 w383]
                frame False {
                  n246 = local read "Auto"() -> (w359:bool)
                  n247 = case shown="False" w359 {
                    tunnel: w358 -> [_ w367]
                    tunnel: w357 -> [_ w366]
                    tunnel: w356 -> [_ w365]
                    tunnel: w355 -> [_ w364]
                    tunnel: w354 -> [_ w363]
                    frame False {
                      n248 = invoke on="Vx" class="DigNum (strict)" method="Reinit To Default"() -> ()  [unwired: 3 in, 3 out]
                    }
                    frame True {
                      n249 = local read "Position(m)"() -> (w361:dbl)
                      n250 = local read "Set X(m)"() -> (w360:dbl)
                      n251 = Not Equal?(x=w360, y=w361) -> (x != y?=w362:bool)
                      n252 = case shown="True" w362 {
                        tunnel: w367 -> [_ w379]
                        tunnel: w366 -> [_ w378]
                        tunnel: w365 -> [_ w377]
                        tunnel: w364 -> [_ w376]
                        tunnel: w363 -> [_ w375]
                        tunnel: w360 -> [_ _]
                        frame False {
                        }
                        frame True {
                          n253 = local read "Layers"() -> (w371:dbl)
                          n254 = local read "Count"() -> (w372:dbl)
                          n255 = control-ref of="Auto"() -> (w373:refnum<vi>)
                          n256 = control-ref of="Vx"() -> (w374:refnum<vi>)
                          n257 = local read "delay"() -> (w369:dbl)
                          n258 = control-ref of="Set X(m)"() -> (w368:refnum<vi>)
                          n259 = Less?(x=w372, y=w371) -> (x < y?=w370:bool)
                          n260 = call "speed control.vi"("flag"=w370, "Power"=w376, "Speed"=w374, "Pos"=w375, "Dest"=w368, "Enable 2"=w373, "delay"=w369, "Set Speed"=w377, "Enable1"=w373, "Deceletration"=w378, "Accletration"=w379) -> ()
                        }
                      }
                    }
                  }
                }
                frame True {
                  n261 = local read "Position(m)"() -> (w382:dbl)
                  n262 = local read "Set X(m)"() -> (w380:dbl)
                  n263 = Not Equal?(x=w382, y=w380) -> (x != y?=w381:bool)
                  n264 = case shown="True" w381 {
                    tunnel: w387 -> [_ w398]
                    tunnel: w386 -> [_ w397]
                    tunnel: w385 -> [_ w396]
                    tunnel: w384 -> [_ w395]
                    tunnel: w383 -> [_ w394]
                    frame False {
                    }
                    frame True {
                      n265 = control-ref of="Forward"() -> (w392:refnum<vi>)
                      n266 = local read "delay"() -> (w389:dbl)
                      n267 = control-ref of="Backward"() -> (w393:refnum<vi>)
                      n268 = control-ref of="Vx"() -> (w391:refnum<vi>)
                      n269 = control-ref of="Set X(m)"() -> (w388:refnum<vi>)
                      n270 = call "speed control.vi"("flag"=FALSE ("repeat"), "Power"=w396, "Speed"=w391, "Pos"=w395, "Dest"=w388, "Enable 2"=w393, "delay"=w389, "Set Speed"=w394, "Enable1"=w392, "Deceletration"=w397, "Accletration"=w398) -> ()
                    }
                  }
                }
              }
            }
            frame True {
              n271 = local read "Set X(m)"() -> (w402:dbl)
              n272 = local read "Position(m)"() -> (w401:dbl)
              n273 = Select(t=0.0, s=w405, f=w402) -> (s? t:f=w399:dbl)
              n274 = local write "Set X(m)"(w399) -> ()
              n275 = Not Equal?(x=w399, y=w401) -> (x != y?=w400:bool)
              n276 = case shown="True" w400 {
                tunnel: w408 -> [_ w420]
                tunnel: w407 -> [_ w419]
                tunnel: w404 -> [_ w414]
                tunnel: w403 -> [_ w413]
                frame False {
                  w409 = FALSE ("Home")
                  n277 = local write "Home"(w409) -> ()
                  n278 = local write "Rapid"(w409) -> ()
                }
                frame True {
                  n279 = control-ref of="Home"() -> (w416:refnum<vi>)
                  n280 = control-ref of="Set X(m)"() -> (w410:refnum<vi>)
                  n281 = control-ref of="Rapid"() -> (w415:refnum<vi>)
                  n282 = control-ref of="Vx"() -> (w418:refnum<vi>)
                  n283 = call "speed control.vi"("flag"=FALSE ("repeat"), "Power"=w414, "Speed"=w418, "Pos"=w413, "Dest"=w410, "Enable 2"=w415, "delay"="delay", "Set Speed"=1.0, "Enable1"=w416, "Deceletration"=w419, "Accletration"=w420) -> ()
                }
              }
            }
          }
        }
        n284 = stacked-sequence {
          frame #0 {
            n285 = Divide(x=1.0, y=97.0) -> (x/y=w320:dbl)
            n286 = Divide(x=1.0, y=190.0) -> (x/y=w326:dbl)
            n287 = property on="Tension\nChart" class="WFChart (strict)"("History Data"=cluster{"Speed":dbl, "Vr":dbl}[] [], "XScale.Maximum"=5.0 ("X Scale.Range:Maximum"), "XScale.Multiplier"=w326) -> ()  [unwired: 2 in, 2 out]
            n288 = property on="Rotation" class="WFChart (strict)"("History Data"=cluster{"Vs":dbl, "Vx":dbl}[] [], "XScale.Maximum"=5.0 ("X Scale.Range:Maximum"), "XScale.Multiplier"=w320) -> ()  [unwired: 2 in, 2 out]
          }
          frame #1 {
            n289 = while {
              stop <- w332 continue-if-true
              n290 = local read "Power"() -> (w332:bool)
              n291 = local read "Vs"() -> (w331:dbl)
              n292 = local read "Vx"() -> (w330:dbl)
              n293 = Bundle("Vs"=w331, "Vx"=w330) -> (→"Rotation":cluster{"Vs":dbl, "Vx":dbl})  [unwired: 1 in]
              n294 = Wait (ms)(milliseconds to wait=u32 10) -> ()  [unwired: 1 out]
            }
          }
        }
      }
    }
  }
  n295 = invoke on="Power" class="Bool (strict)" method="Reinit To Default"() -> ()  [unwired: 3 in, 3 out]
  n296 = invoke on="Trajectory" class="LabVIEW 3D Graph (strict)" method="Reinit To Default"() -> ()  [unwired: 3 in, 3 out]
  n297 = invoke on="Tension\nChart" class="WFChart (strict)" method="Reinit To Default"() -> ()  [unwired: 3 in, 3 out]
